vi "Swerve Begin.vi"   [LabVIEW 2020]
uses:
  <vilib>/Rock Robotics/WPI/ThirdParty/JAS_Junk/TrajLib/Trajectory_Library.lvlib
  Robot Global Data.vi
  <vilib>/Rock Robotics/WPI/Gyro/WPI_GyroAnalogOpen.vi
  <vilib>/Rock Robotics/SystemInterfaces/AI/FPGA_AIGyroChannel.ctl
types:
  T1 = typedef "FPGA_AIGyroChannel.ctl" = enum8{"AI 0", "AI 1", "Invalid"}
  T2 = typedef "Trajectory_Library.lvlib/ROTATION2D.ctl" = cluster{"VALUE":dbl, "COS":dbl, "SIN":dbl}
  T3 = typedef "Trajectory_Library.lvlib/SWERVE_DRIVE_MODULE_STATE.ctl" = cluster{"Speed":dbl, "Angle":T2}
  T4 = typedef "Trajectory_Library.lvlib/SWERVE_DRIVE_MODULE_POSITION.ctl" = cluster{"Distance":dbl, "Angle":T2, "P":bool}
  T5 = typedef "Trajectory_Library.lvlib/TRANSLATION2D.ctl" = cluster{"X":dbl, "Y":dbl}
  T6 = typedef "Trajectory_Library.lvlib/SWERVE_DRIVE_KINEMATICS.ctl" = cluster{"NumModules":i32, "InverseKinematics":T7, "ForwardKinematics":T7, "Modules":T5[], "PrevCoR":T5, "SavedModuleStates":T3[]}
  T7 = typedef "NI_Matrix.lvlib/RealMatrix.ctl" = dbl[][]
  T8 = typedef "Trajectory_Library.lvlib/POSE2D.ctl" = cluster{"TRANSLATION":T5, "ROTATION":T2}
  T9 = typedef "Trajectory_Library.lvlib/SWERVE_DRIVE_ODOMETRY.ctl" = cluster{"POSE":T8, "GyroOffset":T2, "PreviousAngle":T2, "PrevModulePositions":T4[], "NumModules":i32}
  T10 = typedef "WPI_GyroDevRef.ctl" = cluster{"DevStatus":errorcluster, "Analog Channel":T11, "Gain (VoltsPerDegree/Second)":dbl, "Gyro Type":enum16{"Analog", "XRS450"}, "Handle":i32, "SPI Bus":T12, "Device Found":bool, "Sample Rate":dbl, "Calibrate On Open":bool, "Offset":dbl}
  T11 = typedef "FPGA_AIChannel.ctl" = enum8{"AI 0", "AI 1", "AI 2", "AI 3", "AI MXP 0", "AI MXP 1", "AI MXP 2", "AI MXP 3", "Invalid"}
  T12 = typedef "spi_bus.ctl" = enum16{"SPI On-Board, CS0", "SPI On-Board, CS1", "SPI On-Board, CS2", "SPI On-Board, CS3", "SPI MXP", "Invalid"}
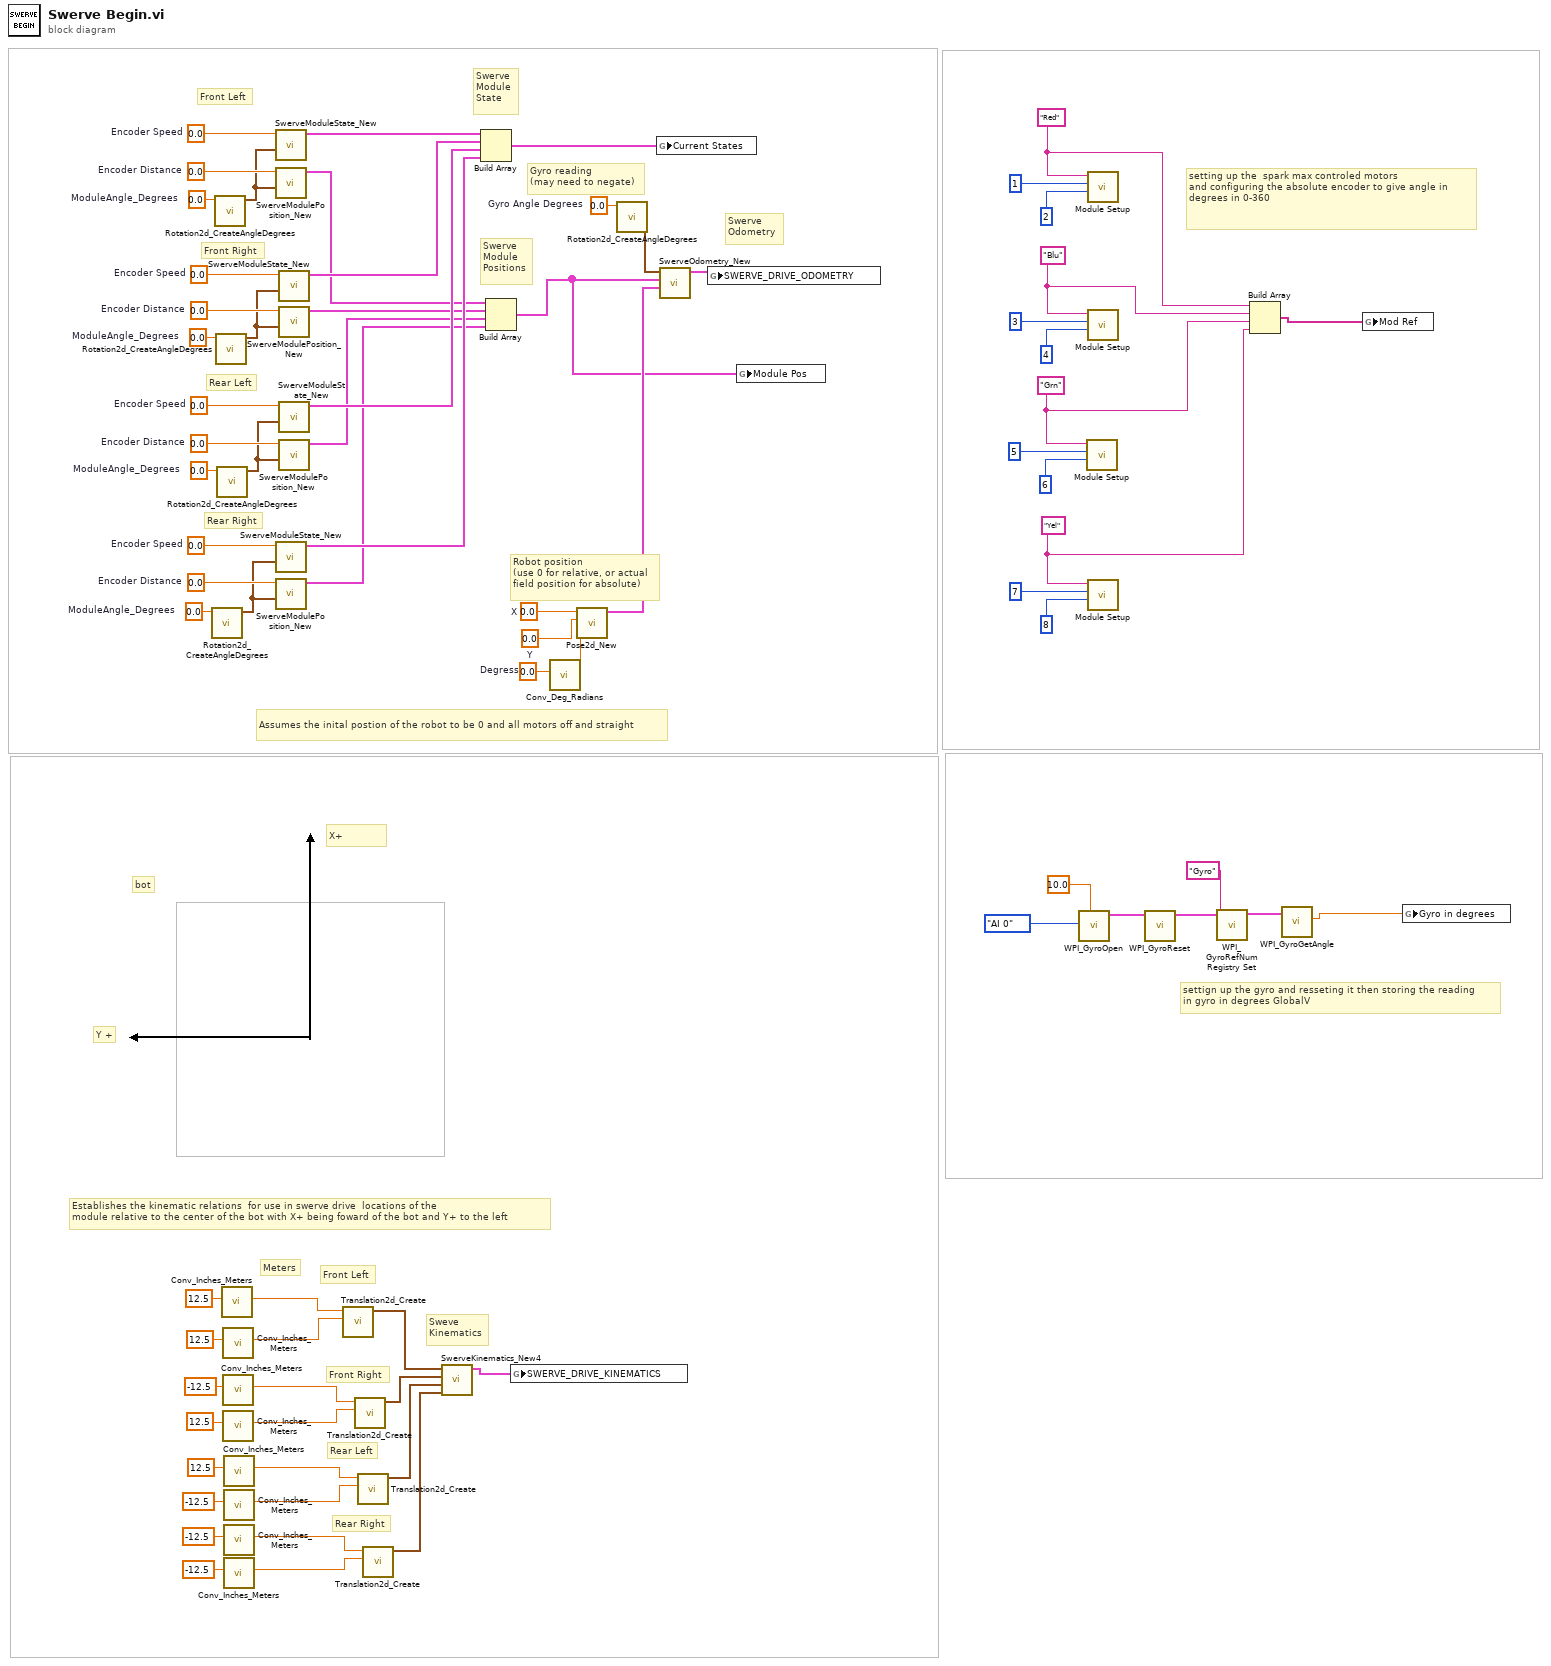
[diagram p0: block diagram]
diagram:
  w74 = "Yel" ("string")
  w73 = "Grn" ("string")
  w72 = "Blu" ("string")
  w71 = "Red" ("string")
  w46 = 0.0  # Encoder Distance
  w47 = 0.0  # Encoder Distance
  w48 = 0.0  # Encoder Distance
  w50 = 0.0  # Encoder Distance
  w54 = 0.0  # ModuleAngle_Degrees
  w55 = 0.0  # Encoder Speed
  w56 = 0.0  # ModuleAngle_Degrees
  w57 = 0.0  # Encoder Speed
  w58 = 0.0  # ModuleAngle_Degrees
  w59 = 0.0  # Encoder Speed
  w61 = 0.0  # ModuleAngle_Degrees
  w62 = 0.0  # Encoder Speed
  w8 = 0.0  # Degress
  w9 = 0.0  # X
  w10 = 0.0  # Y
  w13 = 0.0  # Gyro Angle Degrees
  # "Establishes the kinematic relations  for use in swerve drive  locations of the \nmodule relative to the center of the bot with X+ being foward of the bot and Y+ to the left"
  # "Y +"
  # "X+"
  # "bot"
  # "Assumes the inital postion of the robot to be 0 and all motors off and straight"
  # "Swerve\nModule\nPositions"
  # "Front Left"
  # "Swerve\nModule\nState"
  # "Rear Right"
  # "Rear Left"
  # "Front Right"
  # "settign up the gyro and resseting it then storing the reading \nin gyro in degrees GlobalV"
  # "setting up the  spark max controled motors\nand configuring the absolute encoder to give angle in \ndegrees in 0-360"
  # "Swerve\nOdometry"
  # "Robot position\n(use 0 for relative, or actual \nfield position for absolute)"
  # "Gyro reading\n(may need to negate)"
  # "Meters"
  # "Sweve\nKinematics"
  # "Rear Right"
  # "Rear Left"
  # "Front Right"
  # "Front Left"
  n1 = call <vilib>:"Rotation2d_CreateAngleDegrees.vi"("Angle_Degrees"=w54) -> ("ROTATION"=w39:T2)  [unwired: 10 in]
  n2 = call <vilib>:"Rotation2d_CreateAngleDegrees.vi"("Angle_Degrees"=w61) -> ("ROTATION"=w42:T2)  [unwired: 10 in]
  n3 = call <vilib>:"Rotation2d_CreateAngleDegrees.vi"("Angle_Degrees"=w58) -> ("ROTATION"=w41:T2)  [unwired: 10 in]
  n4 = call <vilib>:"Rotation2d_CreateAngleDegrees.vi"("Angle_Degrees"=w56) -> ("ROTATION"=w40:T2)  [unwired: 10 in]
  n5 = call <vilib>:"Conv_Inches_Meters.vi"("INCH"=12.5) -> ("Meters"=w32:dbl)  [unwired: 10 in]
  n6 = call <vilib>:"Conv_Inches_Meters.vi"("INCH"=12.5) -> ("Meters"=w24:dbl)  [unwired: 10 in]
  n7 = call <vilib>:"Conv_Inches_Meters.vi"("INCH"=-12.5) -> ("Meters"=w33:dbl)  [unwired: 10 in]
  n8 = call <vilib>:"Conv_Inches_Meters.vi"("INCH"=12.5) -> ("Meters"=w34:dbl)  [unwired: 10 in]
  n9 = call <vilib>:"Conv_Inches_Meters.vi"("INCH"=12.5) -> ("Meters"=w35:dbl)  [unwired: 10 in]
  n10 = call <vilib>:"Conv_Inches_Meters.vi"("INCH"=-12.5) -> ("Meters"=w36:dbl)  [unwired: 10 in]
  n11 = call <vilib>:"Conv_Inches_Meters.vi"("INCH"=-12.5) -> ("Meters"=w37:dbl)  [unwired: 10 in]
  n12 = call <vilib>:"Conv_Inches_Meters.vi"("INCH"=-12.5) -> ("Meters"=w38:dbl)  [unwired: 10 in]
  n13 = call <vilib>:"SwerveModuleState_New.vi"("ROTATION"=w42, "Speed"=w62) -> ("SWERVE_DRIVE_MODULE_STATE"=w60:T3)  [unwired: 9 in]
  n14 = call <vilib>:"SwerveModulePosition_New.vi"("ROTATION"=w42, "Distance"=w50) -> ("SWERVE_DRIVE_MODULE_POSITION"=w49:T4)  [unwired: 9 in]
  n15 = call <vilib>:"SwerveModuleState_New.vi"("ROTATION"=w39, "Speed"=w55) -> ("SWERVE_DRIVE_MODULE_STATE"=w51:T3)  [unwired: 9 in]
  n16 = call <vilib>:"SwerveModulePosition_New.vi"("ROTATION"=w39, "Distance"=w46) -> ("SWERVE_DRIVE_MODULE_POSITION"=w43:T4)  [unwired: 9 in]
  n17 = call <vilib>:"SwerveModuleState_New.vi"("ROTATION"=w41, "Speed"=w59) -> ("SWERVE_DRIVE_MODULE_STATE"=w53:T3)  [unwired: 9 in]
  n18 = call <vilib>:"SwerveModulePosition_New.vi"("ROTATION"=w41, "Distance"=w48) -> ("SWERVE_DRIVE_MODULE_POSITION"=w45:T4)  [unwired: 9 in]
  n19 = call <vilib>:"SwerveModuleState_New.vi"("ROTATION"=w40, "Speed"=w57) -> ("SWERVE_DRIVE_MODULE_STATE"=w52:T3)  [unwired: 9 in]
  n20 = call <vilib>:"SwerveModulePosition_New.vi"("ROTATION"=w40, "Distance"=w47) -> ("SWERVE_DRIVE_MODULE_POSITION"=w44:T4)  [unwired: 9 in]
  n21 = call <vilib>:"Translation2d_Create.vi"("Y"=w24, "X"=w32) -> ("TRANSLATION"=w5:T5)  [unwired: 9 in]
  n22 = call <vilib>:"Translation2d_Create.vi"("Y"=w34, "X"=w33) -> ("TRANSLATION"=w4:T5)  [unwired: 9 in]
  n23 = call <vilib>:"Translation2d_Create.vi"("Y"=w36, "X"=w35) -> ("TRANSLATION"=w3:T5)  [unwired: 9 in]
  n24 = call <vilib>:"Translation2d_Create.vi"("Y"=w38, "X"=w37) -> ("TRANSLATION"=w2:T5)  [unwired: 9 in]
  n25 = call <vilib>:"SwerveKinematics_New4.vi"("wheel 3"=w2, "wheel 2"=w3, "wheel 1"=w4, "wheel 0"=w5) -> ("SWERVE_DRIVE_KINEMATICS"=w6:T6)  [unwired: 7 in]
  n26 = Build Array(w60, w53, w52, w51) -> (w63:T3[])
  n27 = Build Array(w49, w45, w44, w43) -> (w1:T4[])
  n28 = global write "Robot Global Data.vi" "SWERVE_DRIVE_KINEMATICS"(w6) -> ()
  n29 = call <vilib>:"Conv_Deg_Radians.vi"("Degress"=w8) -> ("Radians"=w11:dbl)  [unwired: 10 in]
  n30 = call <vilib>:"Pose2d_New.vi"("Heading"=w11, "Y"=w10, "X"=w9) -> ("out POSe"=w7:T8)  [unwired: 8 in]
  n31 = call <vilib>:"Rotation2d_CreateAngleDegrees.vi"("Angle_Degrees"=w13) -> ("ROTATION"=w12:T2)  [unwired: 10 in]
  n32 = global write "Robot Global Data.vi" "Current States"(w63) -> ()
  n33 = call <vilib>:"SwerveOdometry_New.vi"("InitialPose"=w7, "Module Positions"=w1, "gyroAngle"=w12) -> ("SWERVE_DRIVE_ODOMETRY"=w14:T9)  [unwired: 8 in]
  n34 = global write "Robot Global Data.vi" "SWERVE_DRIVE_ODOMETRY"(w14) -> ()
  n35 = global write "Robot Global Data.vi" "Module Pos"(w1) -> ()
  n36 = call-poly <vilib>:"WPI_GyroOpen.vi"("Calibration Time (s)"=10.0, "Analog Channel"=FPGA_AIGyroChannel."AI 0") -> ("GyroDevRef"=w18:T10)  [unwired: 7 in, 2 out]
  n37 = call "Module Setup.vi"("Vel ID"=u8 6 ("Device Number"), "Rot ID"=u8 5 ("Device Number"), "Mod Des"=w73) -> ()  [unwired: 9 in]
  n38 = call "Module Setup.vi"("Vel ID"=u8 2 ("Device Number"), "Rot ID"=u8 1 ("Device Number"), "Mod Des"=w71) -> ()  [unwired: 9 in]
  n39 = call "Module Setup.vi"("Vel ID"=u8 4 ("Device Number"), "Rot ID"=u8 3 ("Device Number"), "Mod Des"=w72) -> ()  [unwired: 9 in]
  n40 = call "Module Setup.vi"("Vel ID"=u8 8 ("Device Number"), "Rot ID"=u8 7 ("Device Number"), "Mod Des"=w74) -> ()  [unwired: 9 in]
  n41 = call <vilib>:"WPI_GyroReset.vi"("GyroDevRef"=w18) -> ("GyroDevRef"=w19:T10)  [unwired: 9 in, 1 out]
  n42 = call <vilib>:"WPI_GyroRefNum Registry Set.vi"("refnum name"="Gyro", "GyroDevRef"=w19) -> ("GyroDevRef"=w20:T10)  [unwired: 8 in, 1 out]
  n43 = Build Array(w71, w72, w73, w74) -> (w75:string[])
  n44 = call <vilib>:"WPI_GyroGetAngle.vi"("GyroDevRef"=w20) -> ("Angle"=w21:dbl)  [unwired: 6 in, 4 out]
  n45 = global write "Robot Global Data.vi" "Mod Ref"(w75) -> ()
  n46 = global write "Robot Global Data.vi" "Gyro in degrees"(w21) -> ()
